vi "PC_Main_Helmet.vi"() -> ()   [LabVIEW 2017]
doc: "This is the PC VI for the autonomous visor cycling (AVC) helmet. For user interaction (GUI), initializing and receiving shared variables, acquiring video stream from the helmet camera, and conducting image processing. By Andrew Shacker, Ning Xuan Tan, and Xander White. Spring 2018."
uses:
  <vilib>/vision/NI_Vision_Development_Module.lvlib
  <vilib>/Utility/miscctls.llb/LVRectTypeDef.ctl
panel:
  in  "Retract":bool
  in  "stop":bool
  in  "Knob":i32(knob) scale=0.0..2.0
  out "Visor Deployed":bool
  in  "Tab Control":T1(tab)
  out "Image Out":T2(plugin-control)
  in  "Motion Estimation":T3={"Level"=4, "Iterations"=5, "Window"=17, "Threshold"=0.01} caption="Options"
  out "LKP Point":cluster{"X":sgl, "Y":sgl}
  out "Prev Frame":cluster{"X":sgl, "Y":sgl}
  out "Matches":i32
  out "IMAQ Cluster":T4={"Score"=1.1006787, "Frame Rate"=31.76130895091434, "Color"=16711930}
  in  "Pitch/Roll Limits":T5
  out "XYZ Cluster":T6
  out "Acceleration":T6(graph)
  out "Pitch/Roll 3D Visualization":refnum<vi>(3d-picture)
  in  "Velocity Threshold (mph)":dbl(slide) scale=0.0..200.0
  out "Distance (ft.)":dbl(graph)
  in  "Minimum Distance from Car (ft)":dbl(slide) scale=0.0..20.0
  out "Distance (ft.)":dbl
  out "Instructions":string
  out "Right":bool
  out "High Turn Rate":bool
  out "Left":bool
  # "Autonomous Visor Cycling Helmet"
  # "Ning Xuan Tan, Andrew Shacker, Xander White"
  # "Rear Vehicle"
  # "Visor"
  # "Stop"
  # "Settings"
  # "Vehicle Detection"
  # "Settings"
  # "Settings"
  # "Settings"
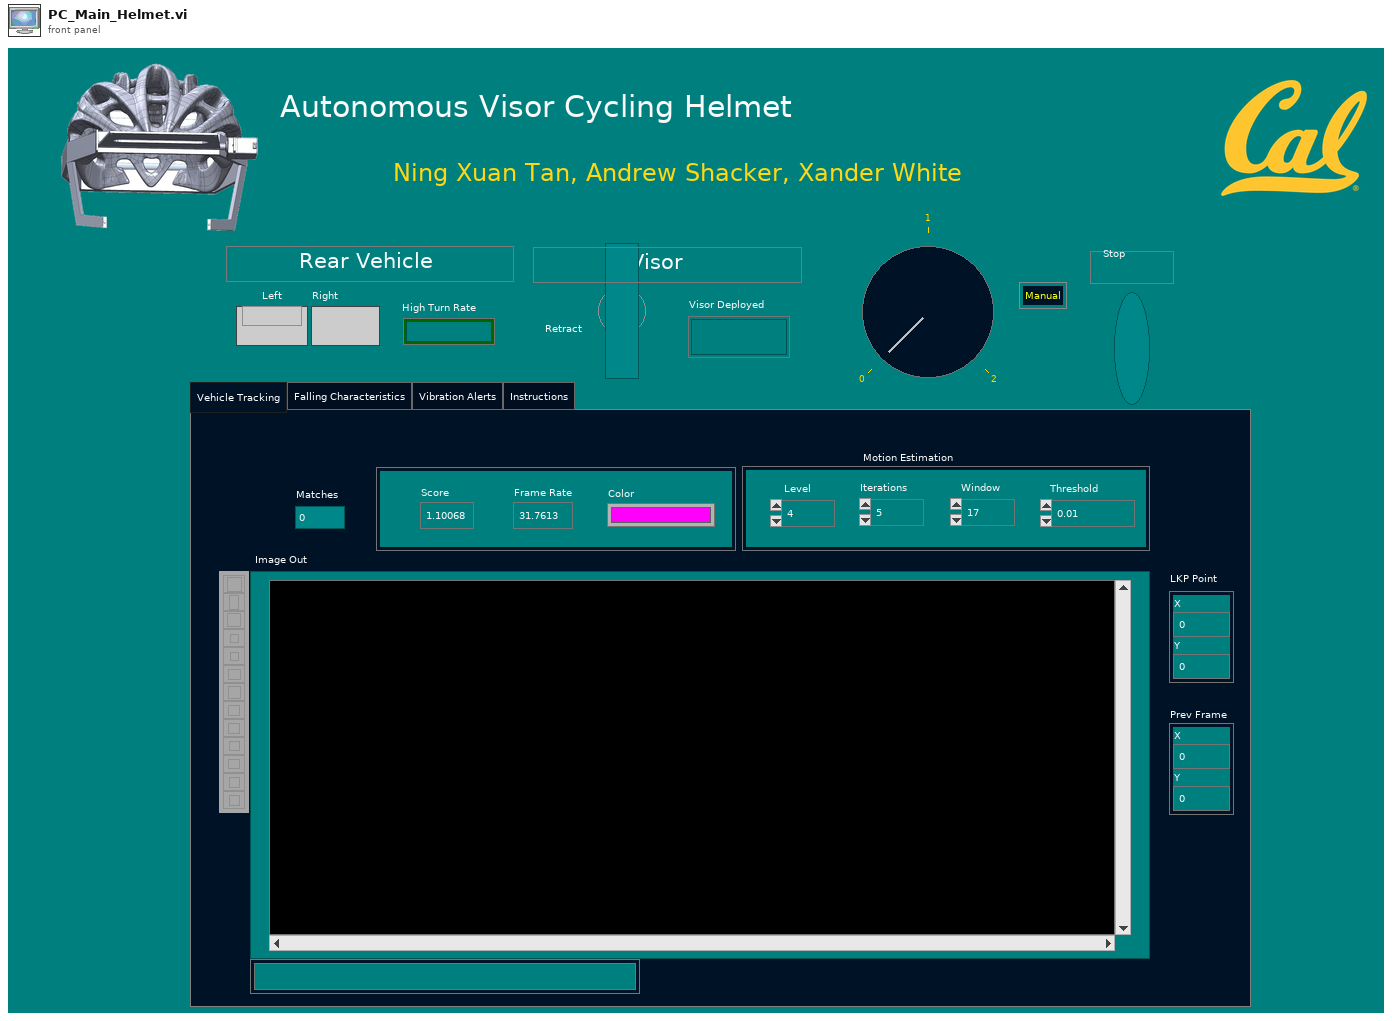
[diagram p1: front panel]
types:
  T1 = enum32{"Vehicle Tracking", "Falling Characteristics", "Vibration Alerts", "Instructions"}
  T2 = typedef "IMAQ Image.ctl" = refnum<image>
  T3 = cluster{"Level":i32, "Iterations":i32, "Window":i32, "Threshold":dbl}
  T4 = cluster{"Score":sgl, "Frame Rate":dbl, "Color":u32}
  T5 = cluster{"Min. Pitch Rate (°/s)":dbl, "Min. Roll Angle (°)":dbl, "Min. Pitch Angle (°)":dbl, "Min. Roll Rate (°/s)":dbl}
  T6 = cluster{"X-Axis":dbl, "Y-Axis":dbl, "Z-Axis":dbl}
  T7 = typedef "LVRectTypeDef.ctl" = cluster{"Left":i16, "Top":i16, "Right":i16, "Bottom":i16}
  T8 = typedef "IMAQ GM Match Report.ctl" = cluster{"Position":cluster{"x":sgl, "y":sgl}, "Angle":sgl, "Scale":sgl, "Score":sgl, "Bounding Box":cluster{"x":sgl, "y":sgl}[], "Contrast Reversed":bool, "Occlusion %":sgl, "Template Target Curve Score":sgl, "Target Template Curve Score":sgl, "Correlation Score":sgl}
  T9 = cluster{"Matches (Geometric Matching 2)[0]":T8, "Matches (Geometric Matching 2)[1]":T8, "Matches (Geometric Matching 2)[2]":T8, "Matches (Geometric Matching 2)[3]":T8, "Matches (Geometric Matching 2)[4]":T8, "Matches (Geometric Matching 2)[5]":T8, "Matches (Geometric Matching 2)[6]":T8, "Matches (Geometric Matching 2)[7]":T8, "Matches (Geometric Matching 2)[8]":T8}
  T10 = cluster{"Bounding Box[0]":cluster{"x":sgl, "y":sgl}, "Bounding Box[1]":cluster{"x":sgl, "y":sgl}, "Bounding Box[2]":cluster{"x":sgl, "y":sgl}, "Bounding Box[3]":cluster{"x":sgl, "y":sgl}, "Bounding Box[4]":cluster{"x":sgl, "y":sgl}, "Bounding Box[5]":cluster{"x":sgl, "y":sgl}, "Bounding Box[6]":cluster{"x":sgl, "y":sgl}, "Bounding Box[7]":cluster{"x":sgl, "y":sgl}, "Bounding Box[8]":cluster{"x":sgl, "y":sgl}}
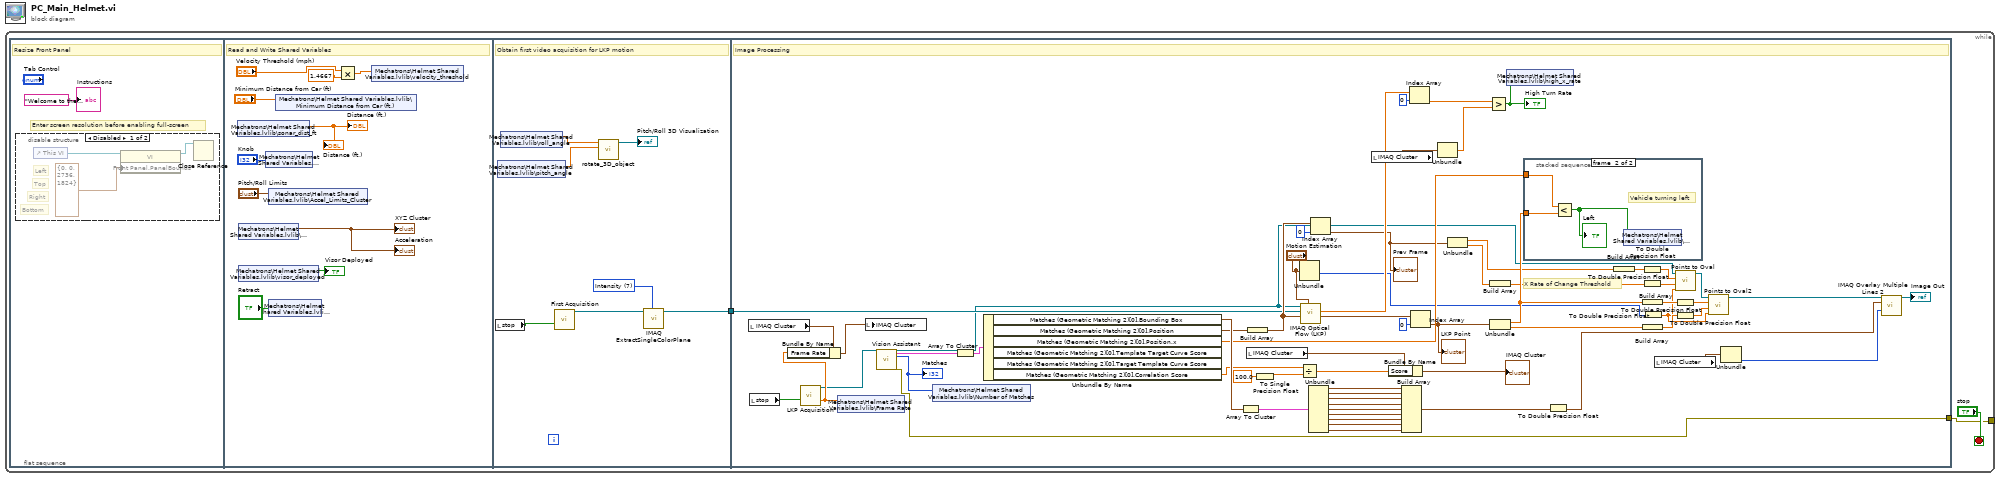
[diagram p0: block diagram]
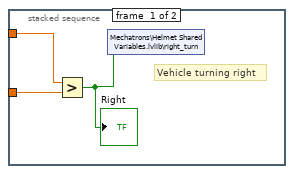
[diagram p3: hidden frame]
diagram:
  n1 = while {
    tunnel: [w1] -> _
    stop <- "stop" stop-if-true
    n2 = flat-sequence {
      tunnel: [w22] -> w2
      tunnel: w2 -> [w33]
      tunnel: [w25] -> w1
      frame #0 {
        # "Enter screen resolution before enabling full-screen"
        # "Resize Front Panel"
        n3 = disable-structure shown="Disabled" {
          frame Disabled {
            # "Bottom"
            # "Right"
            # "Top"
            # "Left"
            n4 = control-ref of="This VI"() -> (w7:refnum<vi>)
            n5 = property class="VI"(reference=w7, "Front Panel.PanelBounds"=T7 {"Left"=0, "Top"=0, "Right"=2736, "Bottom"=1824} ("Front Panel Window:Panel Bounds")) -> (reference out=w5:refnum<vi>)  [unwired: 1 in, 1 out]
            n6 = Close Reference(reference=w5) -> ()  [unwired: 1 in, 1 out]
          }
          frame Enabled {
          }
        }
        "Instructions" <- "Welcome to the Autonomous Visor Cycling Helmet GUI by Ning Xuan Tan, Andrew Shacker, and Xander White, 2018.\n\nGuide\n1. Connect the myRio to WiFi/USB.\n2. Follow the \"Integrating Android Devices with NI Sofware\" tutorial at: http://www.ni.com/example/31558/en/ to use your phone's camera for vehicle detection and tracking.\n*For a quickstart, choose an existing webcam from the Vision Acquisition wizard.\n3. Run the myRio VI labeled \"Main_myRIO_helmet.vi\" from the project tree.\n4. Run this VI, which should enter fullscreen. If only part of the VI is showing, exit the VI and check the resolution constants in the block diagram.\n5. Set your desired settings in each tab above.\n6. Your helmet is ready to use!\n\nModes\nManual: Deploys visor only when button0 on myRIO is pressed.\nAuto: Deploys visor when fall is detected.\nSafe: Deploys visor when fall is detected or vehicle detected and approaching at or within minimum set rate (and range). \n\nPrimary Indicators\nRear Vehicle: Left and Right boolean indicators show which direction the car being tracked by your camera is shifting behind you using motion estimation.\nVisor: Retract will retract the visor if it has been deployed. Visor Deployed shows whether a signal has been sent to the servo to deploy the visor.\n\nCredits\nWe would like to thank the following individuals for their help with our project:\nProf. George Anwar     GSI Drew Sabelhaus     Bola Malek (Triathlete)" ("String")
      }
      frame #1 {
        # "Read and Write Shared Variables"
        n7 = shared-variable "Mechatrons\\Helmet Shared Variables.lvlib\\sonar_dist_ft"() -> (→"Distance (ft.)" →"Distance (ft.)":dbl)  [unwired: 1 in, 1 out]
        n8 = shared-variable "Mechatrons\\Helmet Shared Variables.lvlib\\xyz_accel"() -> (→"XYZ Cluster" →"Acceleration":T6)  [unwired: 1 in, 1 out]
        n9 = shared-variable "Mechatrons\\Helmet Shared Variables.lvlib\\visor_deployed"() -> (→"Visor Deployed":bool)  [unwired: 1 in, 1 out]
        n10 = shared-variable "Mechatrons\\Helmet Shared Variables.lvlib\\Knob"("Knob") -> ()  [unwired: 1 in, 1 out]
        n11 = shared-variable "Mechatrons\\Helmet Shared Variables.lvlib\\Accel_Limits_Cluster"("Pitch/Roll Limits") -> ()  [unwired: 1 in, 1 out]
        n12 = shared-variable "Mechatrons\\Helmet Shared Variables.lvlib\\Retract"("Retract") -> ()  [unwired: 1 in, 1 out]
        n13 = shared-variable "Mechatrons\\Helmet Shared Variables.lvlib\\Minimum Distance from Car (ft.)"("Minimum Distance from Car (ft)") -> ()  [unwired: 1 in, 1 out]
        n14 = Multiply(x="Velocity Threshold (mph)", y=1.4667) -> (x*y=w8:dbl)
        n15 = shared-variable "Mechatrons\\Helmet Shared Variables.lvlib\\velocity_threshold"(w8) -> ()  [unwired: 1 in, 1 out]
      }
      frame #2 {
        w23 = 7 items=["Red", "Green", "Blue", "Hue", "Saturation", "Luminance", "Value", "Intensity"] ("Color Plane")
        # "Obtain first video acquisition for LKP motion"
        n16 = local read "stop"() -> (w21:bool)
        n17 = shared-variable "Mechatrons\\Helmet Shared Variables.lvlib\\pitch_angle"() -> (w20:dbl)  [unwired: 1 in, 1 out]
        n18 = shared-variable "Mechatrons\\Helmet Shared Variables.lvlib\\roll_angle"() -> (w19:dbl)  [unwired: 1 in, 1 out]
        n19 = call "First Acquisition"("Stop (F)"=w21) -> ("Image Out"=w24:T2)  [unwired: 23 in, 3 out]
        n20 = call "rotate_3D_object.vi"("Z (Pitch)"=w20, "X (Roll)"=w19) -> ("3D Picture"=→"Pitch/Roll 3D Visualization":refnum<vi>)  [unwired: 9 in]
        n21 = call "IMAQ ExtractSingleColorPlane"("Color Plane"=w23, "Image Src"=w24) -> ("Image Dst Out"=w22:T2)  [unwired: 8 in, 1 out]
      }
      frame #3 {
        # "X Rate of Change Threshold"
        # "Image Processing"
        n22 = local read "IMAQ Cluster"() -> (w86:T4)
        n23 = local read "stop"() -> (w32:bool)
        n24 = call "LKP Acquisition"("Stop (F)"=w32) -> ("Image Out"=w29:T2, "Frame Rate"=w87:dbl)  [unwired: 23 in, 2 out]
        n25 = Bundle By Name(cluster=w86, "Frame Rate"=w87) -> (w88:T4)
        n26 = shared-variable "Mechatrons\\Helmet Shared Variables.lvlib\\Frame Rate"(w87) -> ()  [unwired: 1 in, 1 out]
        n27 = local write "IMAQ Cluster"(w88) -> ()
        n28 = call "Vision Assistant"("Image In"=w29) -> ("Image Out"=w31:T2, "Matches (Geometric Matching 2)"=w30:T8[], "Number of Matches (Geometric Matching 2)"=w28:i32, "error out"=w25:errorcluster)  [unwired: 23 in]
        "Matches" <- w28
        n29 = shared-variable "Mechatrons\\Helmet Shared Variables.lvlib\\Number of Matches"(w28) -> ()  [unwired: 1 in, 1 out]
        n30 = Array To Cluster(array=w30) -> (cluster=w79:T9)
        n31 = Unbundle By Name(w79) -> ("Matches (Geometric Matching 2)[0].Bounding Box"=w80:cluster{"x":sgl, "y":sgl}[], "Matches (Geometric Matching 2)[0].Position"=w52:cluster{"x":sgl, "y":sgl}, "Matches (Geometric Matching 2)[0].Position.x"=w61:sgl, "Matches (Geometric Matching 2)[0].Correlation Score"=w77:sgl)  [unwired: 2 out]
        n32 = Array To Cluster(array=w80) -> (cluster=w62:T10)
        n33 = local read "IMAQ Cluster"() -> (w82:T4)
        n34 = Build Array(w52) -> (w51:cluster{"x":sgl, "y":sgl}[])
        n35 = To Single Precision Float(number=100.0) -> (single precision float=w76:sgl)
        n36 = Unbundle("Motion Estimation") -> ("Window"=w53:i32)  [unwired: 3 out]
        n37 = Divide(x=w77, y=w76) -> (x/y=w81:sgl)
        n38 = call "IMAQ Optical Flow (LKP)"("Options"="Motion Estimation", "Feature Points In"=w51, "Previous Frame"=w33, "Current Frame"=w31) -> ("Feature Points Out"=w60:cluster{"X":sgl, "Y":sgl}[], "Distance Array"=w75:dbl[])  [unwired: 4 in, 2 out]
        n39 = Unbundle(w62) -> ("Bounding Box[0]"=w72:cluster{"x":sgl, "y":sgl}, "Bounding Box[1]"=w66:cluster{"x":sgl, "y":sgl}, "Bounding Box[2]"=w71:cluster{"x":sgl, "y":sgl}, "Bounding Box[3]"=w65:cluster{"x":sgl, "y":sgl}, "Bounding Box[4]"=w70:cluster{"x":sgl, "y":sgl}, "Bounding Box[5]"=w78:cluster{"x":sgl, "y":sgl}, "Bounding Box[6]"=w69:cluster{"x":sgl, "y":sgl}, "Bounding Box[7]"=w68:cluster{"x":sgl, "y":sgl}, "Bounding Box[8]"=w67:cluster{"x":sgl, "y":sgl})
        n40 = Index Array(array=w51, index=0) -> (element=w50:cluster{"x":sgl, "y":sgl})
        "Prev Frame" <- w50
        n41 = local read "IMAQ Cluster"() -> (w83:T4)
        n42 = Bundle By Name(cluster=w82, "Score"=w81) -> (→"IMAQ Cluster":T4)
        n43 = Build Array(w72, w66, w71, w65, w70, w78, w69, w68, w67) -> (w46:cluster{"x":sgl, "y":sgl}[])
        n44 = Index Array(array=w75, index=0) -> (element=w74:dbl)
        n45 = Index Array(array=w60, index=0) -> (element=w59:cluster{"X":sgl, "Y":sgl})
        "LKP Point" <- w59
        n46 = Unbundle(w83) -> ("Frame Rate"=w84:dbl)  [unwired: 2 out]
        n47 = Unbundle(w50) -> ("x"=w49:sgl, "y"=w48:sgl)
        n48 = Greater?(x=w74, y=w84) -> (0:w73:bool)
        "High Turn Rate" <- w73
        n49 = Build Array(w48) -> (w45:sgl[])
        n50 = Unbundle(w59) -> ("X"=w58:sgl, "Y"=w57:sgl)
        n51 = shared-variable "Mechatrons\\Helmet Shared Variables.lvlib\\high_x_rate"(w73) -> ()  [unwired: 1 in, 1 out]
        n52 = stacked-sequence {
          tunnel: w58 -> [w90 w94]
          tunnel: w61 -> [w91 w93]
          frame #0 {
            # "Vehicle turning right"
            n53 = Greater?(x=w91, y=w90) -> (0:w89:bool)
            "Right" <- w89
            n54 = shared-variable "Mechatrons\\Helmet Shared Variables.lvlib\\right_turn"(w89) -> ()  [unwired: 1 in, 1 out]
          }
          frame #1 {
            # "Vehicle turning left"
            n55 = Less?(x=w93, y=w94) -> (x < y?=w92:bool)
            "Left" <- w92
            n56 = shared-variable "Mechatrons\\Helmet Shared Variables.lvlib\\left_turn"(w92) -> ()  [unwired: 1 in, 1 out]
          }
        }
        n57 = To Double Precision Float(number=w46) -> (double precision float=w64:cluster{"x":dbl, "y":dbl}[])
        n58 = Build Array(w49) -> (w47:sgl[])
        n59 = To Double Precision Float(number=w47) -> (double precision float=w44:dbl[])
        n60 = To Double Precision Float(number=w45) -> (double precision float=w43:dbl[])
        n61 = Build Array(w58) -> (w55:sgl[])
        n62 = Build Array(w57) -> (w56:sgl[])
        n63 = To Double Precision Float(number=w53) -> (double precision float=w38:dbl)
        n64 = local read "IMAQ Cluster"() -> (w85:T4)
        n65 = call "Points to Oval.vi"("Size"=w38, "Y"=w43, "X"=w44, "Image In"=w31) -> ("Image Out"=w42:T2)  [unwired: 7 in]
        n66 = To Double Precision Float(number=w55) -> (double precision float=w41:dbl[])
        n67 = To Double Precision Float(number=w56) -> (double precision float=w40:dbl[])
        n68 = call "Points to Oval2.vi"("Size"=w38, "Y"=w40, "X"=w41, "Image In"=w42) -> ("Image Out"=w39:T2)  [unwired: 7 in]
        n69 = Unbundle(w85) -> ("Color"=w27:u32)  [unwired: 2 out]
        n70 = call "IMAQ Overlay Multiple Lines 2"("Image"=w39, "Line End Points"=w64, "Color"=w27) -> ("Image Out"=→"Image Out":T2)  [unwired: 11 in, 1 out]
      }
    }
  }
